vi "Read.vi"(8 "error in (no error)":errorcluster, 11 "Videoscan in":refnum<class "Videoscan.lvclass">) -> (0 "error out":errorcluster, 1 "timed out?":bool=TRUE, 2 "Data":refnum<class "AbstractData.lvclass">, 3 "Videoscan out":refnum<class "Videoscan.lvclass">)   [LabVIEW 2014, in "Videoscan.lvclass"]
uses:
  Videoscan.lvclass
  Framework/Model/Data/AbstractData/AbstractData.lvclass
  Framework/Model/Data/Data2D/Data2D.lvclass
  Videoscan.lvclass/Videoscan.ctl
  VideoScanLibrary/VideoScanDeviceLibrary.lvclass
  Framework/Interfaces/Observable Actor/Observable Actor.lvclass
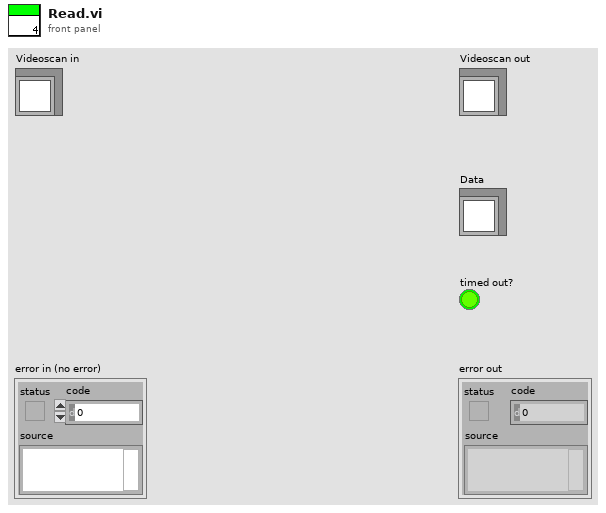
[diagram p1: front panel]
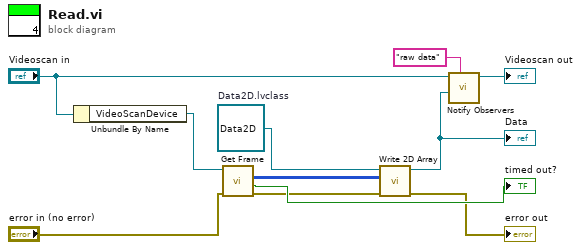
[diagram p0: block diagram]
diagram:
  w9 = refnum<class "Data2D.lvclass"> refnum  # Data2D.lvclass
  n1 = Unbundle By Name("Videoscan in") -> ("VideoScanDevice"=w11:refnum<class "VideoScanDeviceLibrary.lvclass">)
  n2 = call "Get Frame.vi"("error in (no error)"="error in (no error)", "VideoScanCamera in"=w11) -> ("error out"=w7:errorcluster, "error?"=→"timed out?":bool, "Frame"=w1:u16[][])  [unwired: 6 in, 1 out]
  n3 = call "Write 2D Array.vi"("error in (no error)"=w7, "2D Array"=w1, "Data2D in"=w9) -> ("error out"=→"error out":errorcluster, "Data2D out"=w2:refnum<class "Data2D.lvclass">)  [unwired: 7 in]
  "Data" <- w2
  n4 = call "Notify Observers.vi"("name"="raw data", "value"=w2, "Observable Actor in"="Videoscan in") -> ("Observable Actor out"=→"Videoscan out":refnum<class "Videoscan.lvclass">)  [unwired: 7 in, 1 out]
